vi "Get Firmware Version Names.vi"(8 "Error In":errorcluster, 9 "Device Index":u8, 11 "Family Index":T1 items=["National Instruments", "Digilent", "Arduino"]) -> (0 "Error Out":errorcluster, 2 "Firmware Path":path[](array[path]), 3 "Firmware Version Names":string[](array[string]))   [LabVIEW 2014, in "LMH-LINX.lvlib"]
doc: "Get Firmware Version Names for user specified Device Famile and Device ID."
uses:
  <vilib>/MakerHub/LINX/LMH-LINX.lvlib
  <vilib>/MakerHub/LINX/Private/Type Defs/Device Family.ctl
  <vilib>/MakerHub/LINX/Private/Type Defs/All Firmware Data FGV States.ctl
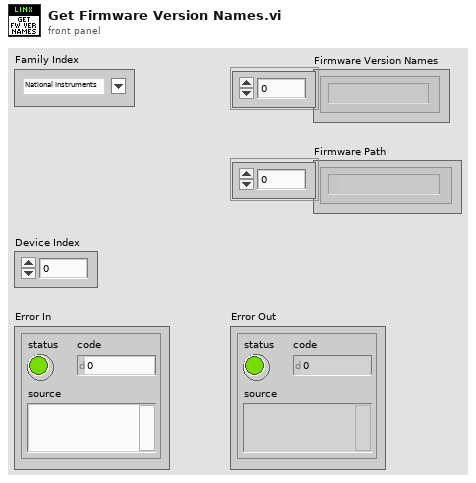
[diagram p1: front panel]
types:
  T1 = typedef "LMH-LINX.lvlib/Device Family.ctl" = u8
  T2 = typedef "LMH-LINX.lvlib/All Firmware Data FGV States.ctl" = enum16{"Set", "Get"}
  T3 = typedef "LMH-LINX.lvlib/Device Firmware.ctl" = cluster{"Firmware Name":string, "Firmware Path":path, "Description":string, "LINX Interface":string, "Flash Util Working Dir":path, "Flash Util Name":string, "Flash Util Args":string, "Flash Timeout (ms)":i32, "Pre-Built Firmware":string, "Build with Arduino IDE":string}
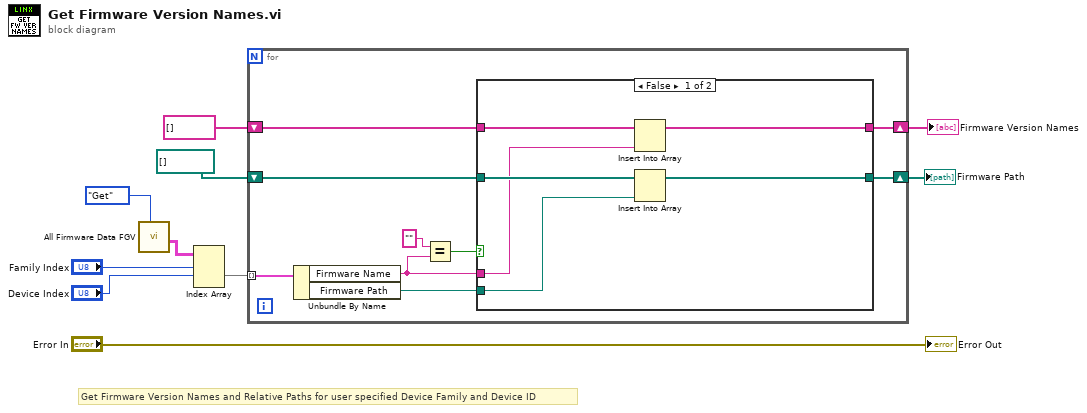
[diagram p0: block diagram]
diagram:
  # "Get Firmware Version Names and Relative Paths for user specified Device Family and Device ID"
  n1 = call <vilib>:"All Firmware Data FGV.vi"("All Firmware Data FGV States"=All_Firmware_Data_FGV_States."Get") -> ("Firmwares"=w8:T3[][][])  [unwired: 7 in, 3 out]
  n2 = Index Array(array=w8, index (dim 0)="Family Index", index (dim 1)="Device Index") -> (element=w5:T3[])  [unwired: 1 in]
  n3 = for {
    tunnel: w5 -> [w19] mode=indexing
    shift-right: [w13] -> w1
    shift-left: path[] [] -> [w14]
    shift-right: [w16] -> w4
    shift-left: string[] [] ("Firmware Version Names") -> [w15]
    n4 = Unbundle By Name(w19) -> ("Firmware Name"=w11:string, "Firmware Path"=w12:path)
    n5 = Equal?(x="", y=w11) -> (x = y?=w17:bool)
    n6 = case shown="False" w17 {
      tunnel: [w22 w27] -> w16
      tunnel: w15 -> [w25 w27]
      tunnel: w14 -> [w24 w26]
      tunnel: [w23 w26] -> w13
      tunnel: w12 -> [w21 _]
      tunnel: w11 -> [w20 _]
      frame False {
        n7 = Insert Into Array(array=w25, new element=w20) -> (w22:string[])  [unwired: 1 in]
        n8 = Insert Into Array(array=w24, new element=w21) -> (w23:path[])  [unwired: 1 in]
      }
      frame True {
      }
    }
  }
  "Firmware Version Names" <- w4
  "Firmware Path" <- w1
  "Error Out" <- "Error In"
